vi "Inspect Transition Manager.vi"(7 "Function":enum16{"Init", "Get Next State"}(ring), 8 "error in (no error)":errorcluster, 11 "Current State":T1) -> (0 "error out":errorcluster, 3 "Next State":T1)   [LabVIEW 2019]
uses:
  Common.llb/IVB State Machine - Transitions Criteria.ctl
  Common.llb/IVB State Machine - Transitions Criteria Function.ctl
  Common.llb/IVB Result Data Types.ctl
  Common.llb/IVB State Machine - Transitions Criteria Result.ctl
  Common.llb/IVB Measure ID.ctl
  Inspect States.ctl
panel:
  in  "Number of States":i32=3
  in  "Transitions":T7(array[cluster])=[{"Name"="default", "Transition Criteria"={"Function"=0, "Type"=enum."Num", "Values"=[], "Mod Bitset"=0}, "Default"=TRUE, "From Index"=0, "To Index"=1, "Priority"=1}, {"Name"="default", "Transition Criteria"={"Function"=0, "Type"=enum."Num", "Values"=[], "Mod Bitset"=0}, "Default"=TRUE, "From Index"=1, "To Index"=2, "Priority"=1}, {"Name"="Loop", "Transition Criteria"={"Function"=0, "Type"=enum."Num", "Values"=[], "Mod Bitset"=0}, "Default"=TRUE, "From Index"=2, "To Index"=0, "Priority"=0}] {"Transition Criteria"."Function" items=["Equal"=0, "Not equal"=1, "Less"=2, "Less or Equal"=3, "Greater"=4, "Greater or Equal"=5, "In Range"=6, "Match Pattern"=7, "NaN"=8, "Result Not Available"=65535]; "Transition Criteria"."Values"."Numeric Constant" format="%.2f"}
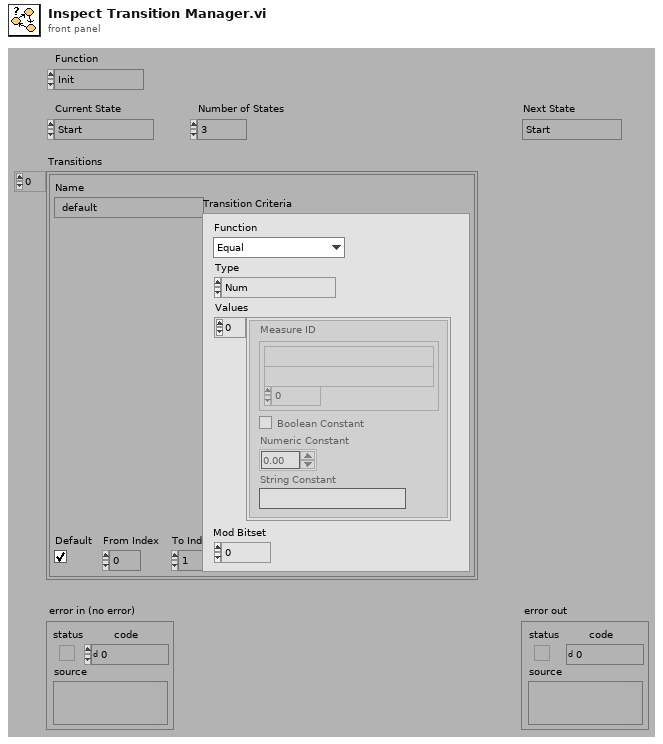
[diagram p1: front panel]
types:
  T1 = typedef "Inspect States.ctl" = enum16{"Start", "Inspect", "End"}
  T2 = typedef "IVB State Machine - Transitions Criteria.ctl" = cluster{"Function":T3, "Type":T4, "Values":T5[], "Mod Bitset":i32}
  T3 = typedef "IVB State Machine - Transitions Criteria Function.ctl" = u16
  T4 = typedef "IVB Result Data Types.ctl" = enum16{"Num", "Bool", "Str", "1D Num", "1D Bool", "1D Str", "Pass/Fail"}
  T5 = typedef "IVB State Machine - Transitions Criteria Result.ctl" = cluster{"Measure ID":T6, "Boolean Constant":bool, "Numeric Constant":dbl, "String Constant":string}
  T6 = typedef "IVB Measure ID.ctl" = cluster{"Step GUID":string, "Result GUID":string, "Index":i32}
  T7 = cluster{"Name":string, "Transition Criteria":T2, "Default":bool, "From Index":i32, "To Index":i32, "Priority":i32}[]
  T8 = cluster{"Name":string, "Transition Criteria":T2, "Default":bool, "From Index":i32, "To Index":i32, "Priority":i32}
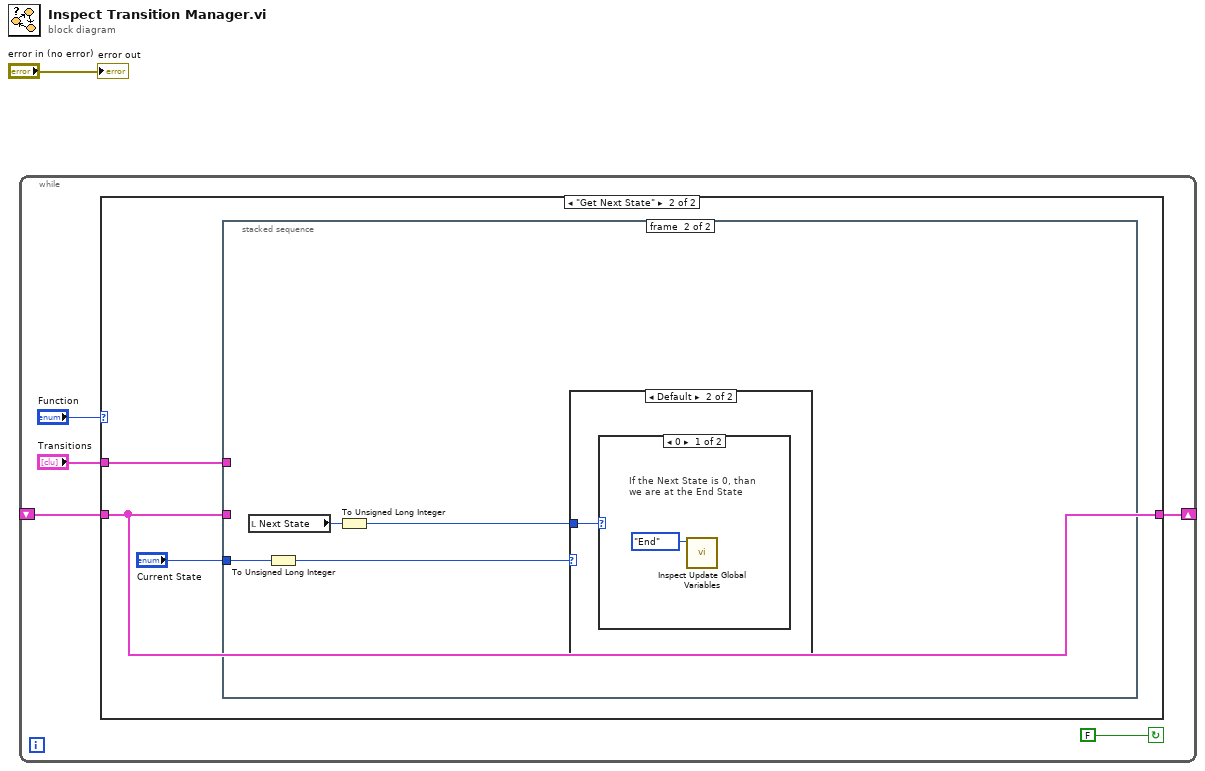
[diagram p0: block diagram]
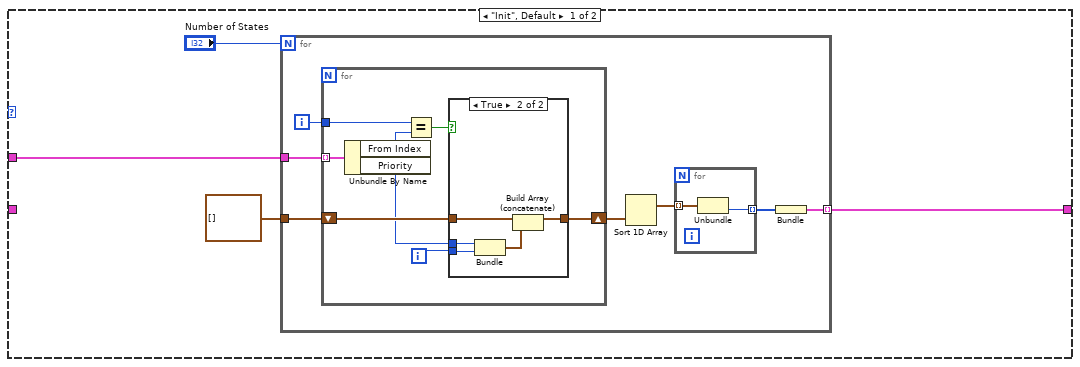
[diagram p2: hidden frame]
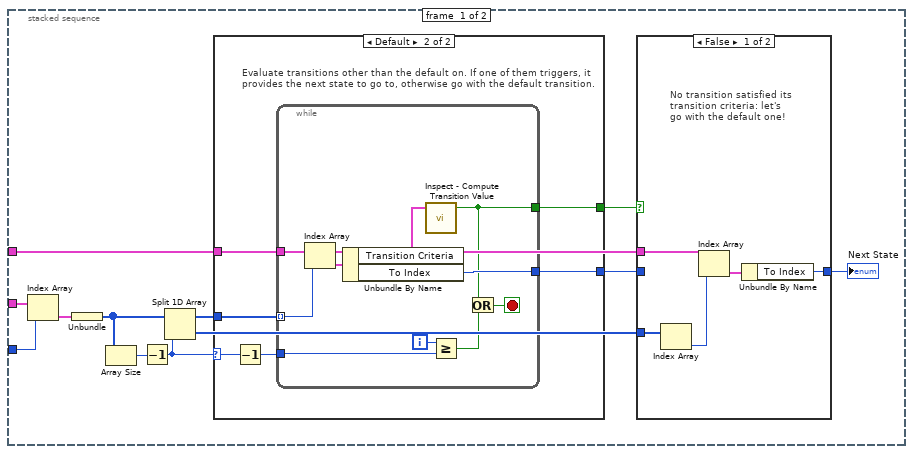
[diagram p4: hidden frame]
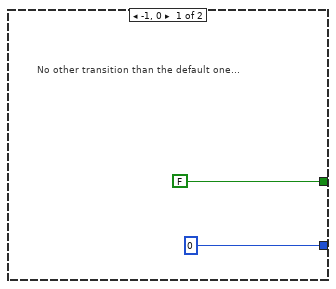
[diagram p6: hidden frame]
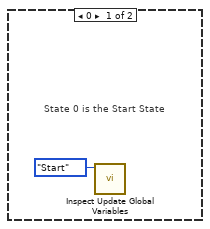
[diagram p7: hidden frame]
diagram:
  n1 = while {
    shift-right: [w3] -> _
    shift-left: _ -> [w6]
    stop <- FALSE continue-if-true
    n2 = case shown="\"Get Next State\"" "Function" {
      tunnel: w6 -> [_ w34]
      tunnel: "Transitions" -> [w9 w36]
      tunnel: [w7 w34] -> w3
      frame "Init", Default {
        n3 = for {
          N: "Number of States" -> [_]
          tunnel: w9 -> [w17]
          tunnel: cluster{"Priority":i32, i32}[] [] -> [w15]
          tunnel: [w11] -> w7 mode=indexing
          i -> [w16]
          n4 = for {
            tunnel: w17 -> [w25] mode=indexing
            shift-right: [w26] -> w14
            shift-left: w15 -> [w27]
            tunnel: w16 -> [w20]
            i -> [w23]
            n5 = Unbundle By Name(w25) -> ("From Index"=w21:i32, "Priority"=w22:i32)
            n6 = Equal?(x=w20, y=w21) -> (x = y?=w24:bool)
            n7 = case shown="True" w24 {
              tunnel: w27 -> [w28 w33]
              tunnel: [w28 w29] -> w26
              tunnel: w23 -> [_ w32]
              tunnel: w22 -> [_ w31]
              frame False {
              }
              frame True {
                n8 = Bundle("Priority"=w31, w32) -> (w30:cluster{"Priority":i32, i32})  [unwired: 1 in]
                n9 = Build Array (concatenate)(w33, w30) -> (w29:cluster{"Priority":i32, i32}[])
              }
            }
          }
          n10 = Sort 1D Array(array=w14) -> (sorted array=w13:cluster{"Priority":i32, i32}[])
          n11 = for {
            tunnel: w13 -> [w19] mode=indexing
            tunnel: [w18] -> w12 mode=indexing
            n12 = Unbundle(w19) -> (w18:i32)  [unwired: 1 out]
          }
          n13 = Bundle(w12) -> (w11:cluster{i32[]})  [unwired: 1 in]
        }
      }
      frame "Get Next State" {
        n14 = stacked-sequence {
          tunnel: w36 -> [w42 _]
          tunnel: "Current State" -> [w41 w76]
          tunnel: w34 -> [w39 _]
          frame #0 {
            n15 = Index Array(array=w39, index=w41) -> (element=w40:cluster{i32[]})
            n16 = Unbundle(w40) -> (w38:i32[])
            n17 = Array Size(array=w38) -> (size(s)=w47:i32)
            n18 = Decrement(x=w47) -> (x-1=w46:i32)
            n19 = Split 1D Array(array=w38, index=w46) -> (first subarray=w48:i32[], second subarray=w43:i32[])
            n20 = case shown="Default" w46 {
              selector: w46 -> [_ w60]
              tunnel: w42 -> [_ w62]
              tunnel: w48 -> [_ w61]
              tunnel: [FALSE w59] -> w45
              tunnel: [0 ("To Index") w58] -> w44
              frame -1, 0 {
                # "No other transition than the default one..."
              }
              frame Default {
                # "Evaluate transitions other than the default on. If one of them triggers, it provides the next state to go to, otherwise go with the default transition."
                n21 = Decrement(x=w60) -> (x-1=w57:i32)
                n22 = while {
                  tunnel: w62 -> [w71]
                  tunnel: w61 -> [w65] mode=indexing
                  tunnel: w57 -> [w69]
                  tunnel: [w68] -> w58
                  tunnel: [w67] -> w59
                  i -> [w64]
                  stop <- w72 stop-if-true
                  n23 = Index Array(array=w71, index=w65) -> (element=w70:T8)
                  n24 = Unbundle By Name(w70) -> ("Transition Criteria"=w66:T2, "To Index"=w68:i32)
                  n25 = call "Inspect - Compute Transition Value.vi"("Transition Criteria"=w66) -> ("Transition Value"=w67:bool)  [unwired: 4 in]
                  n26 = Greater Or Equal?(x=w64, y=w69) -> (x >= y?=w63:bool)
                  n27 = Or(x=w67, y=w63) -> (x .or. y?=w72:bool)
                }
              }
            }
            n28 = case shown="False" w45 {
              tunnel: w44 -> [_ w54]
              tunnel: w42 -> [w52 _]
              tunnel: w43 -> [w53 _]
              tunnel: [w50 w54] -> w37
              frame False {
                # "No transition satisfied its transition criteria: let's go with the default one!"
                n29 = Index Array(array=w53) -> (element=w49:i32)  [unwired: 1 in]
                n30 = Index Array(array=w52, index=w49) -> (element=w51:T8)
                n31 = Unbundle By Name(w51) -> ("To Index"=w50:i32)
              }
              frame True {
                # "A transition was fired as its criteria was satisfied."
              }
            }
            "Next State" <- w37
          }
          frame #1 {
            n32 = local read "Next State"() -> (w74:T1)
            n33 = To Unsigned Long Integer(number=w76) -> (unsigned 32bit integer=w75:u32)
            n34 = To Unsigned Long Integer(number=w74) -> (unsigned 32bit integer=w73:u32)
            n35 = case shown="Default" w75 {
              tunnel: w73 -> [_ w78]
              frame 0 {
                # "State 0 is the Start State"
                n36 = call "Inspect Update Global Variables.vi"("Mode"=enum16{"Start", "End"}."Start") -> ()  [unwired: 11 in]
              }
              frame Default {
                n37 = case shown="0" w78 {
                  frame 0 {
                    # "If the Next State is 0, than we are at the End State"
                    n38 = call "Inspect Update Global Variables.vi"("Mode"=enum16{"Start", "End"}."End") -> ()  [unwired: 11 in]
                  }
                  frame Default {
                  }
                }
              }
            }
          }
        }
      }
    }
  }
  "error out" <- "error in (no error)"
